vi "CHD-simulate-dashboard.vi"() -> ()   [LabVIEW 2019]
uses:
  <vilib>/Rock Robotics/WPI/ThirdParty/JAS_Junk/TrajLib/TypeDef/CHASSIS_SPEEDS.ctl
  <vilib>/Rock Robotics/WPI/ThirdParty/JAS_Junk/TrajLib/TypeDef/POSE2D.ctl
  <vilib>/Rock Robotics/WPI/ThirdParty/JAS_Junk/TrajLib/TypeDef/TRANSLATION2D.ctl
  <vilib>/Rock Robotics/WPI/ThirdParty/JAS_Junk/TrajLib/TypeDef/ROTATION2D.ctl
  Differential_Drive_System/CHD_DRIVE_GLOBALS.vi
  Simulation/CHD_SIM_SIM_Globals.vi
  Trajectory Following/CHD_TRAJECTORY_GLOBALS.vi
  Vision_Interface/CHD_Vision_Globals.vi
  Odometry/CHD_ODOM_GLOBALS.vi
  <vilib>/Rock Robotics/WPI/ThirdParty/ChoreoLib/ChoreoLib.lvlib
  <vilib>/Rock Robotics/WPI/ThirdParty/JAS_Junk/TrajLib/Trajectory_Library.lvlib
panel:
  in  "Tab Control":T1(tab)
  out "Battery Voltage":dbl(graph)
  out "Swerve Motor Demands":T2(graph)
  out "Drive Motor Demands":T2(graph)
  out "Diff Module Devices":T3(array[cluster])
  out "GyroReading_Degreees":dbl format="%15.3f"
  out "Encoder Distances":dbl[](array[numeric]) format="%17.2f"
  out "Encoder Velocities":dbl[](array[numeric]) format="%17.2f"
  out "Motor Demands":dbl[](array[numeric]) format="%17.2f"
  out "Battery Volts":dbl format="%16.2f"
  out "Mod Wheel \nSpeed Dmd":dbl[](array[numeric]) format="%17.3f"
  out "Swerve Drive Motor output":T4(graph)
  out "Drive Wheel Speed M/S":T5(graph)={"LeftSpeed_MperS"=-0.009633185841696038, "RightSpeed_MpserS"=0.013499114310804968}
  out "Drive Speed Error  M/S":T6(graph)={"Mod Wheel Speed Err[0]"=0.009633185841696038, "Mod Wheel Speed Err[1]"=-0.013499114310804968, "Mod Wheel Speed Err[2]"=0.0, "Mod Wheel Speed Err[3]"=0.0}
  out "Closed Loop Control":bool
  out "Orientation Angle Dmd_Rad":dbl format="%17.3f"
  out "Drv Chassis Adj Velocity DmD":T7 {"vOmega" format="%10.3f"; "vY" format="%10.3f"; "vX" format="%10.3f"}
  out "GyroHeading_Radians":dbl format="%17.2f"
  out "Orientation Angle Error_Rad":dbl format="%17.3f"
  out "Orientation Correct CO":dbl format="%17.3f"
  out "Actual Chassis Speed":T7 {"vOmega" format="%10.3f"; "vY" format="%10.3f"; "vX" format="%10.3f"}
  out "Mod Wheel Out":dbl[](array[numeric]) format="%17.3f"
  out "Drive Wheel \nSpeed M/S":dbl[](array[numeric]) format="%17.3f"
  out "Mod Wheel Speed Err":dbl[](array[numeric]) format="%17.3f"
  out "MotorDistances_M":dbl[](array[numeric]) format="%17.2f"
  out "Vision Pose":T8={"TRANSLATION"={"X"=0.0, "Y"=0.0}, "ROTATION"={"VALUE"=0.0, "COS"=1.0, "SIN"=0.0}} {"ROTATION"."SIN" format="%13.4f"; "ROTATION"."COS" format="%13.4f"; "ROTATION"."VALUE" format="%13.4f"; "TRANSLATION"."Y" format="%14.3f"; "TRANSLATION"."X" format="%14.3f"}
  out "Vision\nPose":bool
  out "Trajectory Status":cluster{dbl, dbl, dbl}(graph)
  out "Trajectory Execution \nClosed Loop":bool
  out "Trajectory Error":T11(graph)
  out "Traj_OnTarget":bool
  out "Current Trajectory Odom Pose":T8={"TRANSLATION"={"X"=0.0, "Y"=0.0}, "ROTATION"={"VALUE"=0.0, "COS"=1.0, "SIN"=0.0}} {"ROTATION"."SIN" format="%13.4f"; "ROTATION"."COS" format="%13.4f"; "ROTATION"."VALUE" format="%13.4f"; "TRANSLATION"."Y" format="%14.3f"; "TRANSLATION"."X" format="%14.3f"}
  out "Absolute Odometry \nPose":T8={"TRANSLATION"={"X"=0.0, "Y"=0.0}, "ROTATION"={"VALUE"=0.0, "COS"=1.0, "SIN"=0.0}} {"ROTATION"."SIN" format="%13.4f"; "ROTATION"."COS" format="%13.4f"; "ROTATION"."VALUE" format="%13.4f"; "TRANSLATION"."Y" format="%14.3f"; "TRANSLATION"."X" format="%14.3f"}
  out "Alt ABS Odometry\nPose":T8={"TRANSLATION"={"X"=0.0, "Y"=0.0}, "ROTATION"={"VALUE"=0.0, "COS"=1.0, "SIN"=0.0}} {"ROTATION"."SIN" format="%13.4f"; "ROTATION"."COS" format="%13.4f"; "ROTATION"."VALUE" format="%13.4f"; "TRANSLATION"."Y" format="%14.3f"; "TRANSLATION"."X" format="%14.3f"}
  out "Absolue Trajectory":cluster{dbl[], dbl[]}(graph)
  out "Other Trajectory":cluster{dbl[], dbl[]}(graph)
  out "error out":errorcluster
  # "SIMULATION"
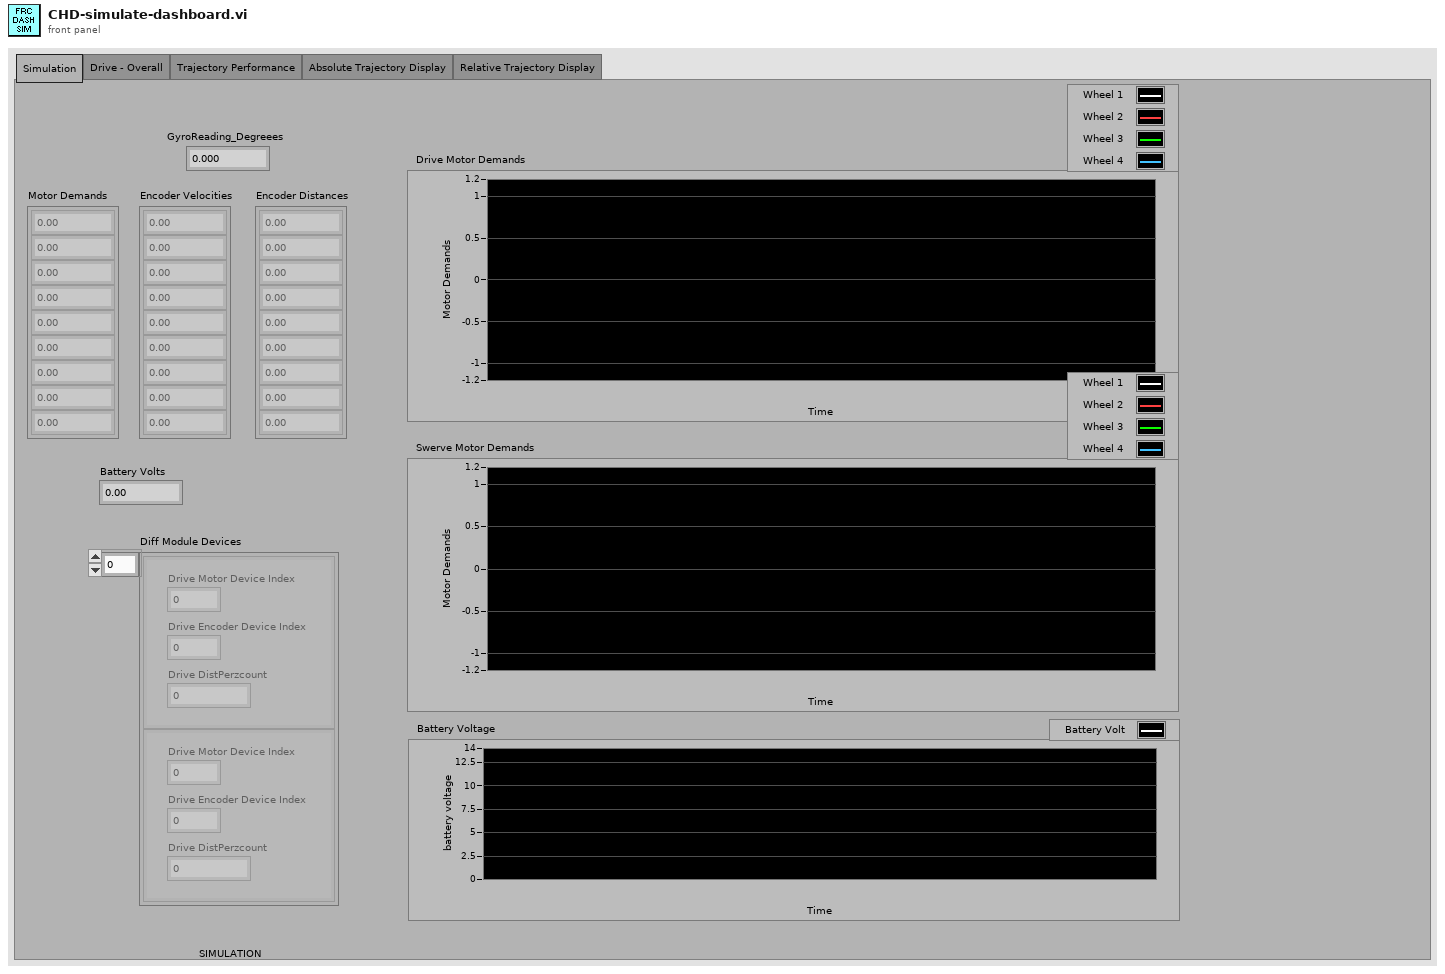
[diagram p1: front panel]
types:
  T1 = enum32{"Simulation", "Drive - Overall", "Trajectory Performance", "Absolute Trajectory Display", "Relative Trajectory Display"}
  T2 = cluster{"Motor Dmd":dbl, "Motor Dmd":dbl, "Motor Dmd":dbl, "Motor Dmd":dbl}
  T3 = cluster{"Drive Motor Device Index":i32, "Drive Encoder Device Index":i32, "Drive DistPerzcount":dbl}[]
  T4 = cluster{"Mod Wheel Out[0]":dbl, "Mod Wheel Out[1]":dbl, "Mod Wheel Out[2]":dbl, "Mod Wheel Out[3]":dbl}
  T5 = cluster{"LeftSpeed_MperS":dbl, "RightSpeed_MpserS":dbl}
  T6 = cluster{"Mod Wheel Speed Err[0]":dbl, "Mod Wheel Speed Err[1]":dbl, "Mod Wheel Speed Err[2]":dbl, "Mod Wheel Speed Err[3]":dbl}
  T7 = typedef "Trajectory_Library.lvlib/CHASSIS_SPEEDS.ctl" = cluster{"vX":dbl, "vY":dbl, "vOmega":dbl}
  T8 = typedef "Trajectory_Library.lvlib/POSE2D.ctl" = cluster{"TRANSLATION":T9, "ROTATION":T10}
  T9 = typedef "Trajectory_Library.lvlib/TRANSLATION2D.ctl" = cluster{"X":dbl, "Y":dbl}
  T10 = typedef "Trajectory_Library.lvlib/ROTATION2D.ctl" = cluster{"VALUE":dbl, "COS":dbl, "SIN":dbl}
  T11 = cluster{"Traj X Err":dbl, "Traj Y Err":dbl, "Traj Heading Err":dbl}
  T12 = cluster{"Traj X Err_FT":dbl, "Traj Y Err_FT":dbl, "Traj Heading Err_DEG":dbl}
  T13 = typedef "ChoreoLib.lvlib/ChoreoTrajectorySwerve.ctl" = cluster{"name":string, "samples":T14[], "splits":i32[], "events":T15[]}
  T14 = typedef "ChoreoLib.lvlib/ChoreoSwerveSample.ctl" = cluster{"timestamp":dbl, "x":dbl, "y":dbl, "heading":dbl, "velocityX":dbl, "velocityY":dbl, "angularVelocity":dbl, "accelX":dbl, "accelY":dbl, "accelAngular":dbl, "forceX":dbl[], "forceY":dbl[]}
  T15 = typedef "ChoreoLib.lvlib/ChoreoEventMarker.ctl" = cluster{"TimeStamp":dbl, "Name":string}
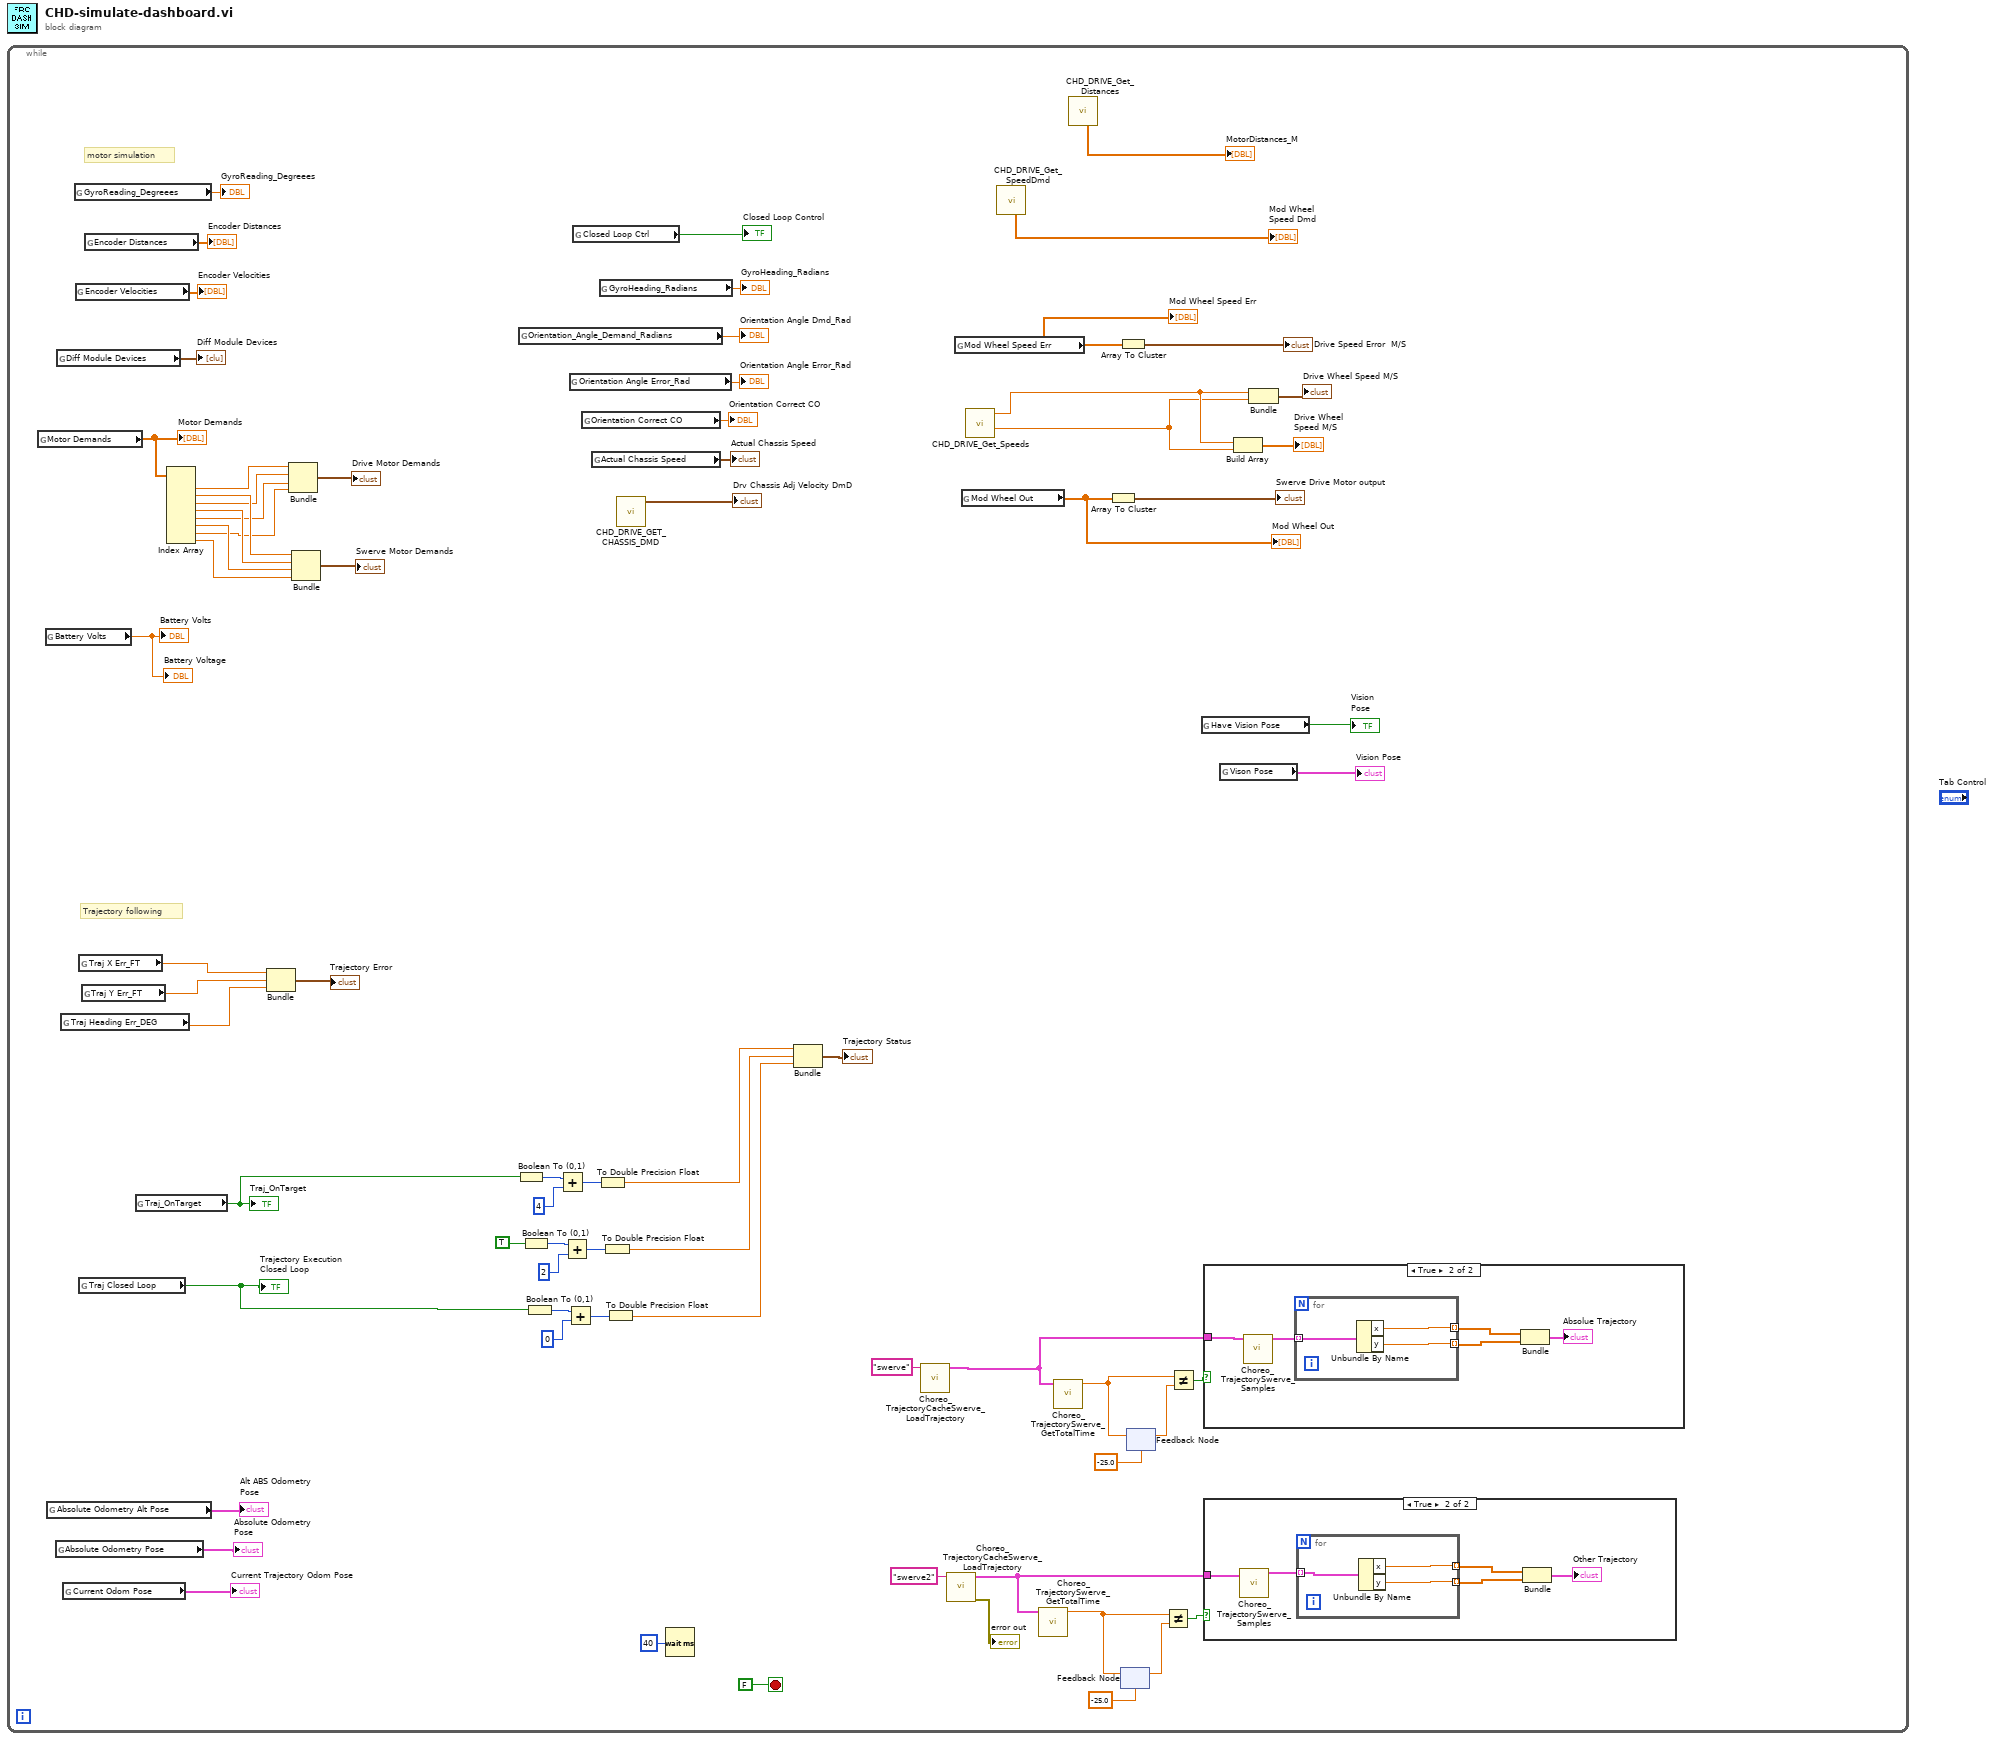
[diagram p0: block diagram]
diagram:
  n1 = while {
    stop <- FALSE stop-if-true
    # "Trajectory following"
    # "motor simulation"
    n2 = global read "CHD_SIM_SIM_Globals.vi" "Motor Demands"() -> (w60:dbl[])
    "Motor Demands" <- w60
    n3 = global read "CHD_SIM_SIM_Globals.vi" "Battery Volts"() -> (→"Battery Volts" →"Battery Voltage":dbl)
    n4 = global read "CHD_ODOM_GLOBALS.vi" "Absolute Odometry Alt Pose"() -> (→"Alt ABS Odometry\nPose":T8)
    n5 = global read "CHD_ODOM_GLOBALS.vi" "Absolute Odometry Pose"() -> (→"Absolute Odometry \nPose":T8)
    n6 = global read "CHD_SIM_SIM_Globals.vi" "Diff Module Devices"() -> (→"Diff Module Devices":T3)
    n7 = global read "CHD_TRAJECTORY_GLOBALS.vi" "Traj Heading Err_DEG"() -> (w47:dbl)
    n8 = global read "CHD_TRAJECTORY_GLOBALS.vi" "Current Odom Pose"() -> (→"Current Trajectory Odom Pose":T8)
    n9 = global read "CHD_SIM_SIM_Globals.vi" "GyroReading_Degreees"() -> (→"GyroReading_Degreees":dbl)
    n10 = global read "CHD_SIM_SIM_Globals.vi" "Encoder Velocities"() -> (→"Encoder Velocities":dbl[])
    n11 = global read "CHD_TRAJECTORY_GLOBALS.vi" "Traj X Err_FT"() -> (w49:dbl)
    n12 = global read "CHD_TRAJECTORY_GLOBALS.vi" "Traj Closed Loop"() -> (w33:bool)
    "Trajectory Execution \nClosed Loop" <- w33
    n13 = global read "CHD_TRAJECTORY_GLOBALS.vi" "Traj Y Err_FT"() -> (w48:dbl)
    n14 = global read "CHD_SIM_SIM_Globals.vi" "Encoder Distances"() -> (→"Encoder Distances":dbl[])
    n15 = global read "CHD_TRAJECTORY_GLOBALS.vi" "Traj_OnTarget"() -> (w45:bool)
    "Traj_OnTarget" <- w45
    n16 = Index Array(array=w60) -> (element #1=w59:dbl, element #2=w58:dbl, element #3=w57:dbl, element #4=w56:dbl, element #5=w55:dbl, element #6=w54:dbl, element #7=w53:dbl, element #8=w52:dbl)  [unwired: 8 in]
    n17 = Bundle("Traj X Err_FT"=w49, "Traj Y Err_FT"=w48, "Traj Heading Err_DEG"=w47) -> (→"Trajectory Error":T12)  [unwired: 1 in]
    n18 = Bundle("Motor Dmd"=w59, "Motor Dmd"=w57, "Motor Dmd"=w55, "Motor Dmd"=w53) -> (→"Drive Motor Demands":T2)  [unwired: 1 in]
    n19 = Bundle("Motor Dmd"=w58, "Motor Dmd"=w56, "Motor Dmd"=w54, "Motor Dmd"=w52) -> (→"Swerve Motor Demands":T2)  [unwired: 1 in]
    n20 = Boolean To (0,1)(Boolean=w45) -> (0, 1=w43:i16)
    n21 = global read "CHD_DRIVE_GLOBALS.vi" "Orientation_Angle_Demand_Radians"() -> (→"Orientation Angle Dmd_Rad":dbl)
    n22 = Boolean To (0,1)(Boolean=TRUE) -> (0, 1=w40:i16)
    n23 = Boolean To (0,1)(Boolean=w33) -> (0, 1=w36:i16)
    n24 = Add(x=w43, y=i16 4) -> (x+y=w42:i16)
    n25 = Add(x=w40, y=i16 2) -> (x+y=w39:i16)
    n26 = Add(x=w36, y=i16 0) -> (x+y=w35:i16)
    n27 = global read "CHD_DRIVE_GLOBALS.vi" "Orientation Angle Error_Rad"() -> (→"Orientation Angle Error_Rad":dbl)
    n28 = global read "CHD_DRIVE_GLOBALS.vi" "Closed Loop Ctrl"() -> (→"Closed Loop Control":bool)
    n29 = global read "CHD_DRIVE_GLOBALS.vi" "Orientation Correct CO"() -> (→"Orientation Correct CO":dbl)
    n30 = global read "CHD_DRIVE_GLOBALS.vi" "Actual Chassis Speed"() -> (→"Actual Chassis Speed":T7)
    n31 = To Double Precision Float(number=w42) -> (double precision float=w44:dbl)
    n32 = global read "CHD_DRIVE_GLOBALS.vi" "GyroHeading_Radians"() -> (→"GyroHeading_Radians":dbl)
    n33 = To Double Precision Float(number=w39) -> (double precision float=w37:dbl)
    n34 = To Double Precision Float(number=w35) -> (double precision float=w32:dbl)
    n35 = call "CHD_DRIVE_GET_CHASSIS_DMD.vi"() -> ("Drv Chassis Velocity DmD"=→"Drv Chassis Adj Velocity DmD":T7)  [unwired: 11 in]
    n36 = Wait (ms)(milliseconds to wait=u32 40) -> ()  [unwired: 1 out]
    n37 = Bundle(w44, w37, w32) -> (→"Trajectory Status":cluster{dbl, dbl, dbl})  [unwired: 1 in]
    n38 = call <vilib>:"Choreo_TrajectoryCacheSwerve_LoadTrajectory.vi"("TrajectoryName"="swerve") -> ("ChoreoTrajectorySwerve"=w12:T13)  [unwired: 9 in, 1 out]
    n39 = call <vilib>:"Choreo_TrajectoryCacheSwerve_LoadTrajectory.vi"("TrajectoryName"="swerve2") -> ("error out"=→"error out":errorcluster, "ChoreoTrajectorySwerve"=w9:T13)  [unwired: 9 in]
    n40 = global read "CHD_DRIVE_GLOBALS.vi" "Mod Wheel Speed Err"() -> (w28:dbl[])
    "Mod Wheel Speed Err" <- w28
    n41 = global read "CHD_DRIVE_GLOBALS.vi" "Mod Wheel Out"() -> (w25:dbl[])
    "Mod Wheel Out" <- w25
    n42 = call "CHD_DRIVE_Get_Speeds.vi"() -> ("RightSpeed_MpserS"=w5:dbl, "LeftSpeed_MperS"=w6:dbl)  [unwired: 9 in, 1 out]
    n43 = call "CHD_DRIVE_Get_SpeedDmd.vi"() -> ("MotorSpeedDmds_MperSec"=→"Mod Wheel \nSpeed Dmd":dbl[])  [unwired: 9 in, 2 out]
    n44 = call <vilib>:"Choreo_TrajectorySwerve_GetTotalTime.vi"("ChoreoTrajectorySwerve"=w9) -> ("TotalTime"=w13:dbl)  [unwired: 10 in]
    n45 = call <vilib>:"Choreo_TrajectorySwerve_GetTotalTime.vi"("ChoreoTrajectorySwerve"=w12) -> ("TotalTime"=w14:dbl)  [unwired: 10 in]
    n46 = call "CHD_DRIVE_Get_Distances.vi"() -> ("MotorDistances_M"=→"MotorDistances_M":dbl[])  [unwired: 9 in, 2 out]
    n47 = Array To Cluster(array=w25) -> (cluster=→"Swerve Drive Motor output":T4)
    n48 = Array To Cluster(array=w28) -> (cluster=→"Drive Speed Error  M/S":T6)
    n49 = feedback #1(-25.0 ("TotalTime_Sec")) -> (w16:dbl)
    n50 = feedback-in #1(w13) -> ()
    n51 = feedback #2(-25.0 ("TotalTime_Sec")) -> (w19:dbl)
    n52 = feedback-in #2(w14) -> ()
    n53 = Not Equal?(x=w13, y=w16) -> (x != y?=w15:bool)
    n54 = Not Equal?(x=w14, y=w19) -> (x != y?=w18:bool)
    n55 = global read "CHD_Vision_Globals.vi" "Have Vision Pose"() -> (→"Vision\nPose":bool)
    n56 = case shown="True" w15 {
      tunnel: w9 -> [_ w75]
      frame False {
      }
      frame True {
        n57 = call <vilib>:"Choreo_TrajectorySwerve_Samples.vi"("ChoreoTrajectorySwerve"=w75) -> ("samples"=w74:T14[])  [unwired: 10 in]
        n58 = for {
          tunnel: [w81] -> w77 mode=indexing
          tunnel: [w80] -> w78 mode=indexing
          tunnel: w74 -> [w79] mode=indexing
          n59 = Unbundle By Name(w79) -> ("x"=w81:dbl, "y"=w80:dbl)
        }
        n60 = Bundle(w77, w78) -> (→"Other Trajectory":cluster{dbl[], dbl[]})  [unwired: 1 in]
      }
    }
    n61 = case shown="True" w18 {
      tunnel: w12 -> [_ w83]
      frame False {
      }
      frame True {
        n62 = call <vilib>:"Choreo_TrajectorySwerve_Samples.vi"("ChoreoTrajectorySwerve"=w83) -> ("samples"=w82:T14[])  [unwired: 10 in]
        n63 = for {
          tunnel: [w89] -> w85 mode=indexing
          tunnel: [w88] -> w86 mode=indexing
          tunnel: w82 -> [w87] mode=indexing
          n64 = Unbundle By Name(w87) -> ("x"=w89:dbl, "y"=w88:dbl)
        }
        n65 = Bundle(w85, w86) -> (→"Absolue Trajectory":cluster{dbl[], dbl[]})  [unwired: 1 in]
      }
    }
    n66 = global read "CHD_Vision_Globals.vi" "Vison Pose"() -> (→"Vision Pose":T8)
    n67 = Build Array(w6, w5) -> (→"Drive Wheel \nSpeed M/S":dbl[])
    n68 = Bundle("LeftSpeed_MperS"=w6, "RightSpeed_MpserS"=w5) -> (→"Drive Wheel Speed M/S":T5)  [unwired: 1 in]
  }
